vi "RF.vi"(1 "In":variant, 2 "Mode":u32(ring) items=["Open", "Close", "Begin", "End", "Get", "Set"]) -> (0 "Out":variant)   [LabVIEW 2014]
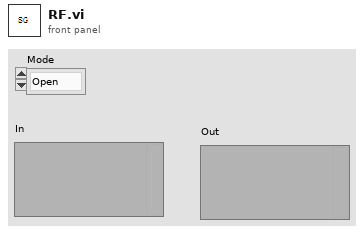
[diagram p1: front panel]
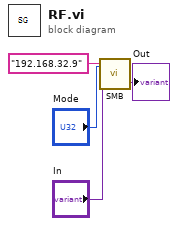
[diagram p0: block diagram]
diagram:
  n1 = call "SMB.vi"("IP"="192.168.32.9", "In"="In", "Mode"="Mode") -> ("Out"=→"Out":variant)
